vi "FRCts20_WebMethods_Events_DELETE.vi"(7 "httpRequestID":u32, 11 "event_name":string) -> ()   [LabVIEW 2014, in "FRCts20_WebMethods.lvlib"]
doc: "<B>DELETE</B> the specified <B>competition</B> resource\n\nhttp://<server address>:<port>/FRCts/competition/<B>competition</B>\n\n{requires authentication}"
uses:
  FRCts20_WebMethods.lvlib
  <vilib>/wsapi/NI_WebServices.lvlib
  Backend/source/VI Source/FRCts20_Backend_API/FRCts20_Backend_API_Event.vi
  Backend/source/VI Source/FRCts20_Backend_API/FRCts20_Backend_API_Event.ctl
  Backend/source/VI Source/FRCts20_Backend_API/FRCts20_Backend_API_Command_Event.ctl
  Backend/source/VI Source/FRCts20_Backend_API/FRCts20_Backend_API_SW.ctl
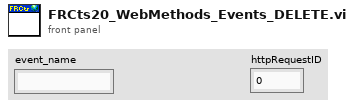
[diagram p1: front panel]
types:
  T1 = typedef "FRCts20_Backend_API.lvlib/FRCts20_Backend_API_Command_Event.ctl" = string
  T2 = typedef "FRCts20_Backend_API.lvlib/FRCts20_Backend_API_Event.ctl" = cluster{"Event Index":u32, "Name":string, "Start Time":timestamp, "End Time":timestamp, "Teams":cluster{"Team Index":u32, "Team Number":u32, "Requests":cluster{"Request Number":u32, "Description":string}[], "Has Open Issue":bool}[], "SWType":T3, "APIReturn":string}
  T3 = typedef "FRCts20_Backend_API.lvlib/FRCts20_Backend_API_SW.ctl" = string
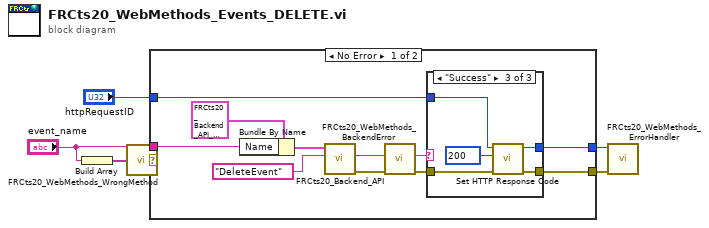
[diagram p0: block diagram]
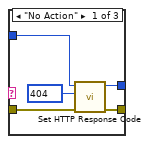
[diagram p2: hidden frame]
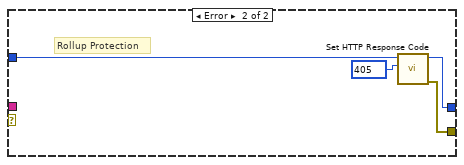
[diagram p4: hidden frame]
diagram:
  n1 = Build Array("event_name") -> (w2:string[])
  n2 = call "FRCts20_WebMethods_WrongMethod.vi"(4:w2) -> (1:w3)  [unwired: 3 in, 1 out]
  n3 = case shown="No Error" w3 {
    tunnel: "httpRequestID" -> [w13 w30]
    tunnel: [w15 w32] -> w5
    tunnel: [w14 w31] -> w4
    tunnel: "event_name" -> [w8 _]
    frame No Error {
      n4 = Bundle By Name(cluster=T2 {"Event Index"=0, "Name"="", "Start Time"=timestamp(0 s since 1904-01-01), "End Time"=timestamp(0 s since 1904-01-01), "Teams"=[], "SWType"="", "APIReturn"=""} ("Event In"), "Name"=w8) -> (w10:T2)
      n5 = call-poly "FRCts20_Backend_API.vi"("Command"=T1 "DeleteEvent", "Event In"=w10) -> ("error out"=w12:errorcluster, "Status"=w9:string)  [unwired: 7 in, 1 out]
      n6 = call "FRCts20_WebMethods_BackendError.vi"("error in (no error)"=w12, "Status"=w9) -> ("error out"=w16:errorcluster, "Status out"=w17:string)  [unwired: 8 in]
      n7 = case shown="\"Success\"" w17 {
        tunnel: w16 -> [w19 w24 w27]
        tunnel: [w22 w24 w26] -> w15
        tunnel: w13 -> [w20 w23 w28]
        tunnel: [w21 w23 w25] -> w14
        frame "No Action" {
          w18 = 404 items=["100"=100, "101"=101, "200"=200, "201"=201, "202"=202, "203"=203, "204"=204, "205"=205, "206"=206, "300"=300, "301"=301, "302"=302, "303"=303, "304"=304, "305"=305, "306"=306, "307"=307, "400"=400, "401"=401, "402"=402, "403"=403, "404"=404, "405"=405, "406"=406, "407"=407, "408"=408, "409"=409, "410"=410, "411"=411, "412"=412, "413"=413, "414"=414, "415"=415, "416"=416, "417"=417, "500"=500, "501"=501, "502"=502, "503"=503, "504"=504, "505"=505] ("response code (200)")
          n8 = call <vilib>:"Set HTTP Response Code.vi"("error in (no error)"=w19, "response code (200)"=w18, "httpRequestID"=w20) -> ("error out"=w22:errorcluster, "httpRequestID out"=w21:u32)  [unwired: 7 in]
        }
        frame "Backend Error", Default {
        }
        frame "Success" {
          w29 = 200 items=["100"=100, "101"=101, "200"=200, "201"=201, "202"=202, "203"=203, "204"=204, "205"=205, "206"=206, "300"=300, "301"=301, "302"=302, "303"=303, "304"=304, "305"=305, "306"=306, "307"=307, "400"=400, "401"=401, "402"=402, "403"=403, "404"=404, "405"=405, "406"=406, "407"=407, "408"=408, "409"=409, "410"=410, "411"=411, "412"=412, "413"=413, "414"=414, "415"=415, "416"=416, "417"=417, "500"=500, "501"=501, "502"=502, "503"=503, "504"=504, "505"=505] ("response code (200)")
          n9 = call <vilib>:"Set HTTP Response Code.vi"("error in (no error)"=w27, "response code (200)"=w29, "httpRequestID"=w28) -> ("error out"=w26:errorcluster, "httpRequestID out"=w25:u32)  [unwired: 7 in]
        }
      }
    }
    frame Error {
      w33 = 405 items=["100"=100, "101"=101, "200"=200, "201"=201, "202"=202, "203"=203, "204"=204, "205"=205, "206"=206, "300"=300, "301"=301, "302"=302, "303"=303, "304"=304, "305"=305, "306"=306, "307"=307, "400"=400, "401"=401, "402"=402, "403"=403, "404"=404, "405"=405, "406"=406, "407"=407, "408"=408, "409"=409, "410"=410, "411"=411, "412"=412, "413"=413, "414"=414, "415"=415, "416"=416, "417"=417, "500"=500, "501"=501, "502"=502, "503"=503, "504"=504, "505"=505] ("response code (200)")
      # "Rollup Protection"
      n10 = call <vilib>:"Set HTTP Response Code.vi"("response code (200)"=w33, "httpRequestID"=w30) -> ("error out"=w32:errorcluster, "httpRequestID out"=w31:u32)  [unwired: 8 in]
    }
  }
  n11 = call "FRCts20_WebMethods_ErrorHandler.vi"("error in"=w5, "LabVIEW Web Service Request"=w4) -> ()  [unwired: 8 in, 2 out]
